vi "Array to Offset and Multiplier.vi"(1 "Array":dbl[](array[numeric])) -> (0 "Offset and Multiplier":T1)   [LabVIEW 2019, in "graph_utilities.lvclass"]
doc: "Given an array, calculate an Offset and Multiplier"
uses:
  graph_utilities.lvclass
  <vilib>/Utility/miscctls.llb/LVOffsetAndMultiplierTypeDef.ctl
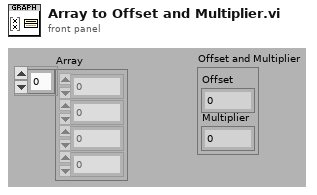
[diagram p1: front panel]
types:
  T1 = typedef "LVOffsetAndMultiplierTypeDef.ctl" = cluster{"Offset":dbl, "Multiplier":dbl}
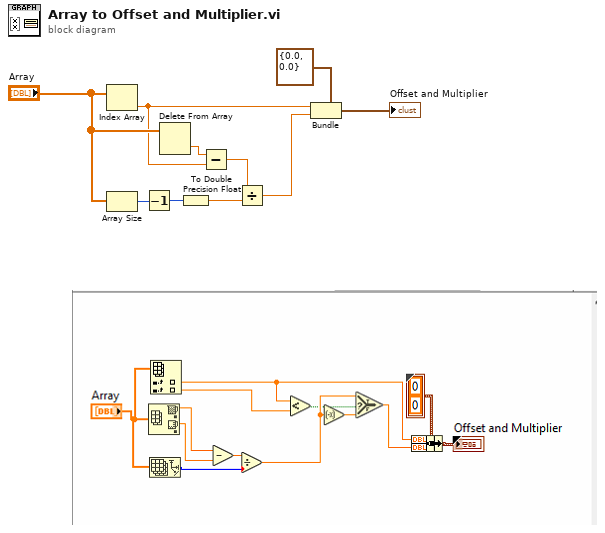
[diagram p0: block diagram]
diagram:
  n1 = Index Array(array="Array") -> (element=w2:dbl)  [unwired: 1 in]
  n2 = Array Size(array="Array") -> (size(s)=w8:i32)
  n3 = Decrement(x=w8) -> (x-1=w6:i32)
  n4 = Delete From Array(array="Array") -> (deleted portion=w3:dbl)  [unwired: 2 in, 1 out]
  n5 = To Double Precision Float(number=w6) -> (double precision float=w7:dbl)
  n6 = Subtract(x=w3, y=w2) -> (x-y=w4:dbl)
  n7 = Divide(x=w4, y=w7) -> (x/y=w1:dbl)
  n8 = Bundle(cluster=T1 {"Offset"=0.0, "Multiplier"=0.0} ("X Scale.Offset and Multiplier"), "Offset"=w2, "Multiplier"=w1) -> (→"Offset and Multiplier":T1)
